vi "InOrderTraverse.vi"(8 "error in (no error)":errorcluster caption="错误输入（无错误）", 9 "Data in":variant, 10 "Method Name":string, 11 "PanelLinkNode 输入":refnum<class "PanelLinkNode.lvclass"> caption="DNL_LabVIEW Object in") -> (0 "error out":errorcluster caption="错误输出", 1 "Data out":variant, 3 "PanelLinkNode 输出":refnum<class "PanelLinkNode.lvclass"> caption="DNL_LabVIEW Object out")   [LabVIEW 2013, in "PanelLinkNode.lvclass"]
uses:
  PanelLinkNode.lvclass
  PanelObject/PanelObject.lvclass
  PanelLinkNode.lvclass/PanelLinkNode.ctl
panel:
  out "数值":i32
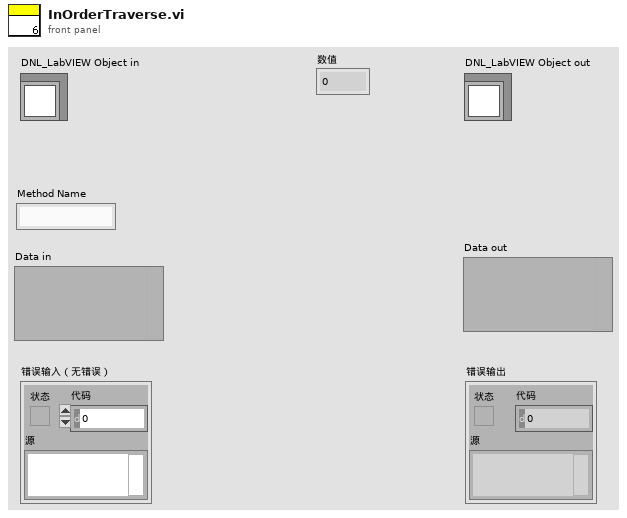
[diagram p1: front panel]
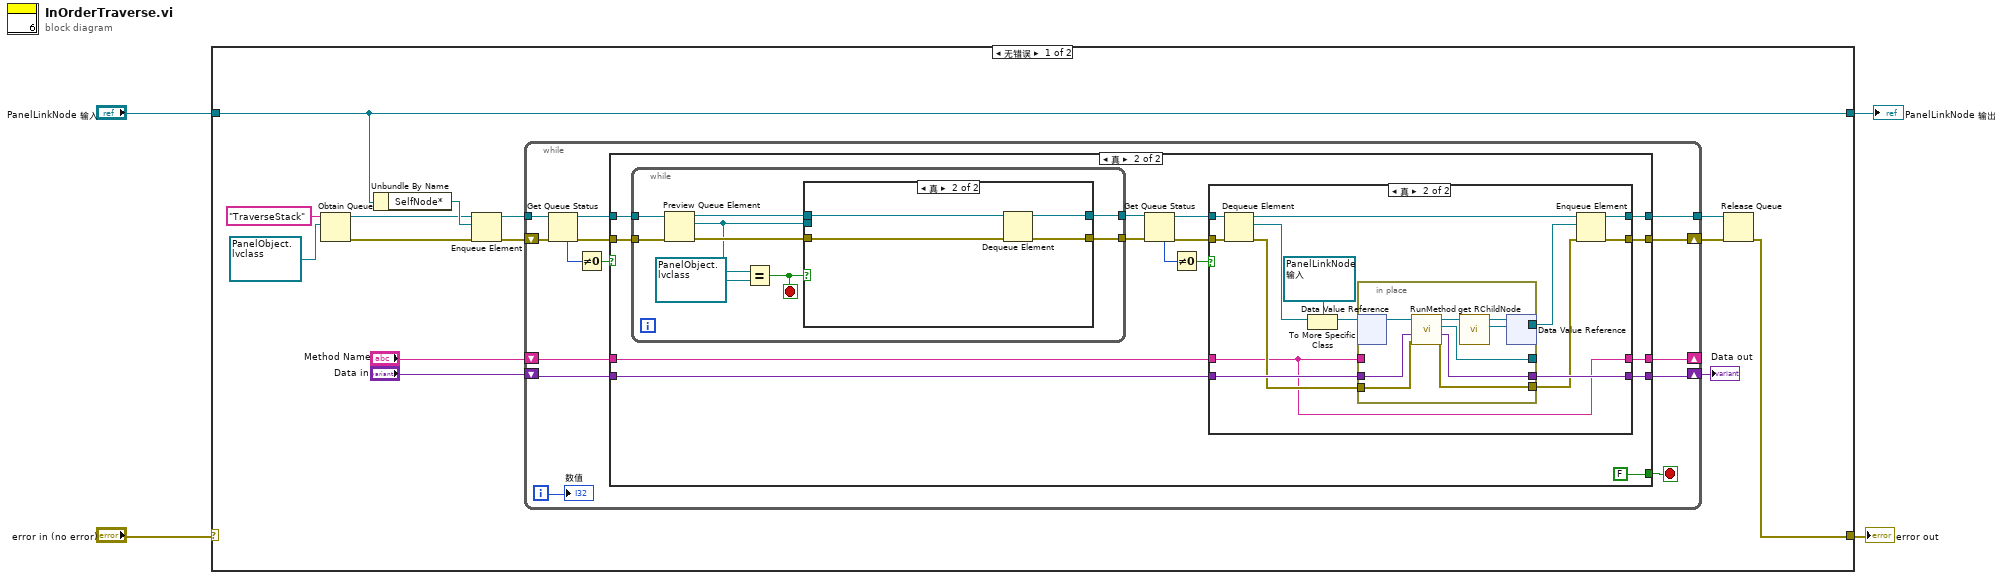
[diagram p0: block diagram]
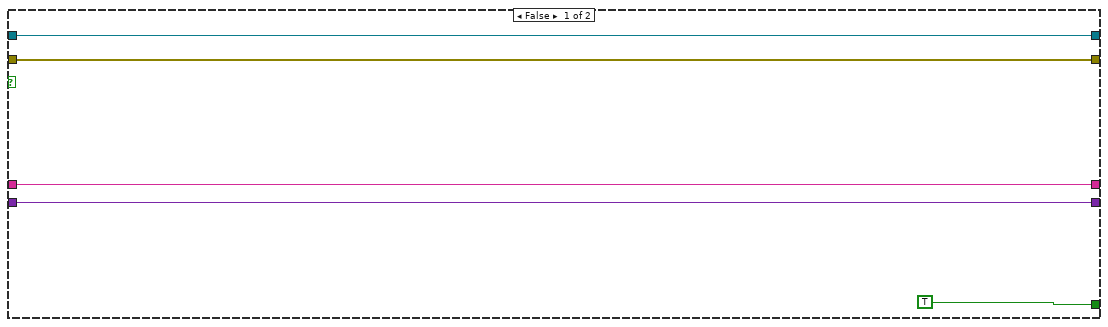
[diagram p2: hidden frame]
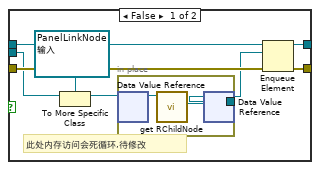
[diagram p4: hidden frame]
diagram:
  n1 = case shown="无错误" "error in (no error)" {
    selector: "error in (no error)" -> [_ w105]
    tunnel: [w9 w105] -> w3
    tunnel: [w6 w104] -> w1
    tunnel: "PanelLinkNode 输入" -> [w6 w104]
    frame No Error {
      n2 = Obtain Queue(name (unnamed)="TraverseStack" ("名称（未命名）"), element data type=refnum<data-value> refnum ("ParentNode*")) -> (queue out=w15:refnum<queue>, error out=w14:errorcluster)  [unwired: 3 in, 1 out]
      n3 = Unbundle By Name(w6) -> ("SelfNode*"=w16:refnum<data-value>)
      n4 = Enqueue Element(queue=w15, element=w16, error in (no error)=w14) -> (queue out=w13:refnum<queue>, error out=w12:errorcluster)  [unwired: 1 in, 1 out]
      n5 = while {
        tunnel: w13 -> [w30]
        tunnel: [w25] -> w11
        shift-right: [w19] -> _
        shift-left: "Method Name" -> [w23]
        shift-right: [w21] -> w5
        shift-left: "Data in" -> [w22]
        shift-right: [w24] -> w10
        shift-left: w12 -> [w31]
        i -> [w20]
        stop <- w32 stop-if-true
        n6 = Get Queue Status(queue=w30, error in (no error)=w31) -> (queue out=w27:refnum<queue>, error out=w26:errorcluster, # elements in queue=w29:i32)  [unwired: 1 in, 5 out]
        n7 = Not Equal To 0?(x=w29) -> (x != 0?=w28:bool)
        n8 = case shown="真" w28 {
          tunnel: [TRUE FALSE] -> w32
          tunnel: w27 -> [w36 w51]
          tunnel: w26 -> [w35 w50]
          tunnel: [w36 w43] -> w25
          tunnel: [w35 w42] -> w24
          tunnel: w23 -> [w34 w41]
          tunnel: w22 -> [w33 w40]
          tunnel: [w34 w39] -> w19
          tunnel: [w33 w38] -> w21
          frame False {
          }
          frame True {
            n9 = while {
              tunnel: w51 -> [w87]
              tunnel: w50 -> [w86]
              tunnel: [w82] -> w48
              tunnel: [w81] -> w47
              stop <- w85 stop-if-true
              n10 = Preview Queue Element(queue=w87, error in (no error)=w86) -> (queue out=w84:refnum<queue>, element=w80:refnum<data-value>, error out=w83:errorcluster)  [unwired: 1 in, 1 out]
              n11 = Equal?(x=w80, y=refnum<data-value> refnum) -> (x = y?=w85:bool)
              n12 = case shown="真" w85 {
                tunnel: w84 -> [w96 w103]
                tunnel: w83 -> [w95 w101]
                tunnel: [w94 w102] -> w82
                tunnel: [w93 w100] -> w81
                tunnel: w80 -> [w90 _]
                frame False {
                  # "此处内存访问会死循环,待修改"
                  n13 = To More Specific Class(target class=refnum<data-value> refnum ("数据值引用"), reference=w90) -> (specific class reference=w89:refnum<data-value>)  [unwired: 1 in, 1 out]
                  n14 = in-place {
                    in-place-border: [w97] -> w92
                    n15 = in-place-dvr #1(w89) -> (w99:refnum<class "PanelLinkNode.lvclass">)  [unwired: 1 out]
                    n16 = call "get RChildNode.vi"("PanelLinkNode输入"=w99) -> ("RChildNode*"=w97:refnum<data-value>, "PanelLinkNode输出"=w98:refnum<class "PanelLinkNode.lvclass">)  [unwired: 8 in, 1 out]
                    n17 = in-place-dvr #1(w98) -> ()  [unwired: 2 out]
                  }
                  n18 = Enqueue Element(queue=w96, element=w92, error in (no error)=w95) -> (queue out=w94:refnum<queue>, error out=w93:errorcluster)  [unwired: 1 in, 1 out]
                }
                frame True {
                  n19 = Dequeue Element(queue=w103, error in (no error)=w101) -> (queue out=w102:refnum<queue>, error out=w100:errorcluster)  [unwired: 1 in, 2 out]
                }
              }
            }
            n20 = Get Queue Status(queue=w48, error in (no error)=w47) -> (queue out=w45:refnum<queue>, error out=w44:errorcluster, # elements in queue=w49:i32)  [unwired: 1 in, 5 out]
            n21 = Not Equal To 0?(x=w49) -> (x != 0?=w46:bool)
            n22 = case shown="真" w46 {
              tunnel: w45 -> [w56 w70]
              tunnel: w44 -> [w55 w69]
              tunnel: [w56 w63] -> w43
              tunnel: [w55 w62] -> w42
              tunnel: w41 -> [w54 w57]
              tunnel: w40 -> [w53 w61]
              tunnel: [w54 w57] -> w39
              tunnel: [w53 w60] -> w38
              frame False {
              }
              frame True {
                n23 = Dequeue Element(queue=w70, error in (no error)=w69) -> (queue out=w68:refnum<queue>, element=w67:refnum<data-value>, error out=w59:errorcluster)  [unwired: 1 in, 1 out]
                n24 = To More Specific Class(target class=refnum<data-value> refnum ("数据值引用"), reference=w67) -> (specific class reference=w65:refnum<data-value>)  [unwired: 1 in, 1 out]
                n25 = in-place {
                  in-place-border: [w78] -> w64
                  in-place-border: w57 -> [_]
                  in-place-border: w61 -> [w75]
                  in-place-border: [w74] -> _
                  in-place-border: [w73] -> w60
                  in-place-border: [w72] -> w58
                  in-place-border: w59 -> [w71]
                  n26 = in-place-dvr #2(w65) -> (w77:refnum<class "PanelLinkNode.lvclass">)  [unwired: 1 out]
                  n27 = call-dynamic "RunMethod.vi"("error in (no error)"=w71, "Data in"=w75, "PanelLinkNode 输入"=w77) -> ("error out"=w72:errorcluster, "Data out"=w73:variant, "vi reference out"=w74:refnum<vi>, "PanelLinkNode 输出"=w76:refnum<class "PanelLinkNode.lvclass">)  [unwired: 4 in, 1 out]
                  n28 = call "get RChildNode.vi"("PanelLinkNode输入"=w76) -> ("RChildNode*"=w78:refnum<data-value>, "PanelLinkNode输出"=w79:refnum<class "PanelLinkNode.lvclass">)  [unwired: 8 in, 1 out]
                  n29 = in-place-dvr #2(w79) -> ()  [unwired: 2 out]
                }
                n30 = Enqueue Element(queue=w68, element=w64, error in (no error)=w58) -> (queue out=w63:refnum<queue>, error out=w62:errorcluster)  [unwired: 1 in, 1 out]
              }
            }
          }
        }
        "数值" <- w20
      }
      "Data out" <- w5
      n31 = Release Queue(queue=w11, error in (no error)=w10) -> (error out=w9:errorcluster)  [unwired: 1 in, 2 out]
    }
    frame Error {
    }
  }
  "error out" <- w3
  "PanelLinkNode 输出" <- w1
